vi "BS find all the tugs.vi"(0 "Image Src":T2, 1 "error in":errorcluster) -> (2 "Tug location array":T1(array[cluster]), 3 "All found?":bool, 4 "error out":errorcluster)   [LabVIEW 2012]
uses:
  <vilib>/vision/Image Controls.llb/IMAQ Image.ctl
  <vilib>/vision/NI_Vision_Development_Module.lvlib
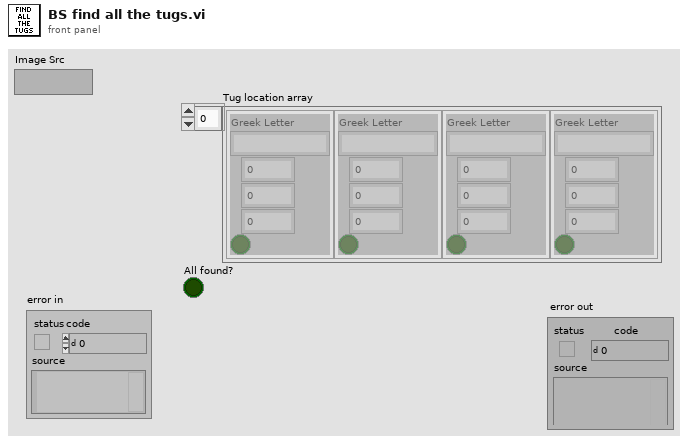
[diagram p1: front panel]
types:
  T1 = cluster{"Greek Letter":string, i16, i16, i16, bool}[]
  T2 = typedef "IMAQ Image.ctl" = refnum<image>
  T3 = enum32{"AutoM", "Close", "Dilate", "Erode", "Gradient", "Gradient in", "Gradient out", "HitMiss", "Open", "PClose", "POpen", "Thick", "Thin"}
  T4 = cluster{"Greek Letter":string, i16, i16, i16, bool}
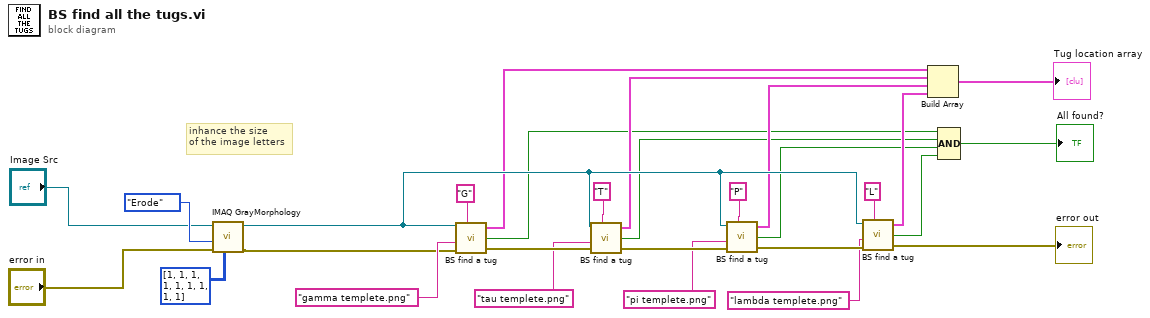
[diagram p0: block diagram]
diagram:
  # "inhance the size \nof the image letters"
  n1 = call "IMAQ GrayMorphology"("Structuring Element"=i32[][] [[1, 1, 1], [1, 1, 1], [1, 1, 1]] ("Structuring Element (Gray Morphology 1)"), "error in (no error)"="error in", "Operation"=T3."Erode" ("Operation (Gray Morphology 1)"), "Image Src"="Image Src") -> ("error out"=w15:errorcluster, "Image Dst Out"=w12:T2)  [unwired: 3 in, 3 out]
  n2 = call "BS find a tug.vi"("Image Path"=w12, "templete path"="gamma templete.png", "error in"=w15, "Greek Letter"="G") -> ("Location"=w10:T4, "Valid?"=w5:bool, "error out"=w26:errorcluster)  [unwired: 1 in]
  n3 = call "BS find a tug.vi"("Image Path"=w12, "templete path"="tau templete.png", "error in"=w26, "Greek Letter"="T") -> ("Location"=w9:T4, "Valid?"=w4:bool, "error out"=w25:errorcluster)  [unwired: 1 in]
  n4 = call "BS find a tug.vi"("Image Path"=w12, "templete path"="pi templete.png", "error in"=w25, "Greek Letter"="P") -> ("Location"=w8:T4, "Valid?"=w3:bool, "error out"=w24:errorcluster)  [unwired: 1 in]
  n5 = call "BS find a tug.vi"("Image Path"=w12, "templete path"="lambda templete.png", "error in"=w24, "Greek Letter"="L") -> ("Location"=w7:T4, "Valid?"=w2:bool, "error out"=→"error out":errorcluster)  [unwired: 1 in]
  n6 = Build Array(w10, w9, w8, w7) -> (→"Tug location array":T1)
  n7 = Compound Arithmetic op=AND(w5, w4, w3, w2) -> (→"All found?":bool)
